vi "Get System Properties.vi"(8 "error in (no error)":errorcluster, 11 "RT System Monitor in":refnum<class "RT System Monitor.lvclass">) -> (0 "error out":errorcluster, 2 "System Health Data":T1 {"Hard Drive Space Used (%)" scale=0.0..100.0}, 3 "RT System Monitor out":refnum<class "RT System Monitor.lvclass">)   [LabVIEW 2017, in "RT System Monitor.lvclass"]
doc: "Poll for CPU usage properties.\nGet total physical memory, hard drive capacity, and total virtual memory.\nPoll for free physical memory, free hard drive space, largest contiguous block of memory, and free virtual memory."
uses:
  RT System Monitor.lvclass
  Shared/System Health Data.ctl
  RT System Monitor.lvclass/RT System Monitor.ctl
  <resource>/objmgr/nicriosae.rc
  <resource>/objmgr/nisysapi.rc
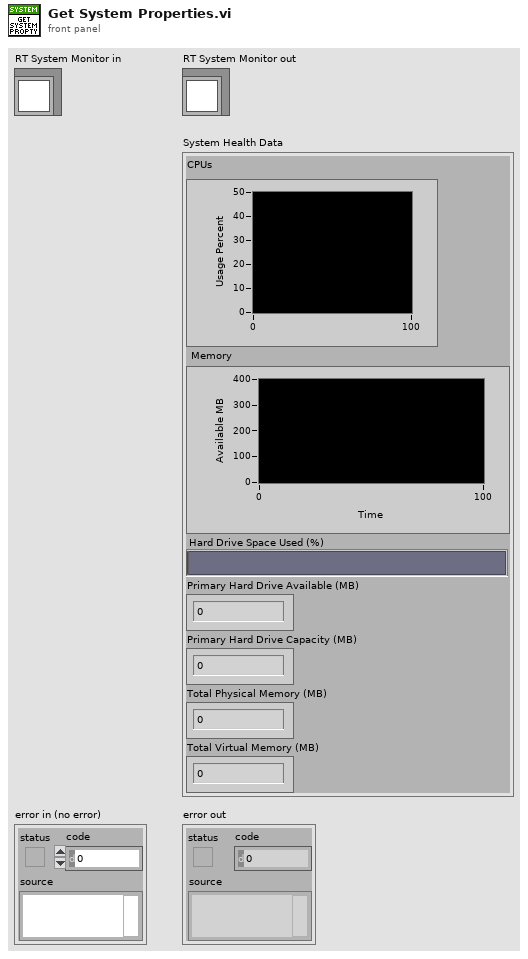
[diagram p1: front panel]
types:
  T1 = typedef "System Health Data.ctl" = cluster{"CPUs":u32[][], "Memory":dbl[][], "Hard Drive Space Used (%)":dbl, "Primary Hard Drive Available (MB)":dbl, "Primary Hard Drive Capacity (MB)":u32, "Total Physical Memory (MB)":u32, "Total Virtual Memory (MB)":u32}
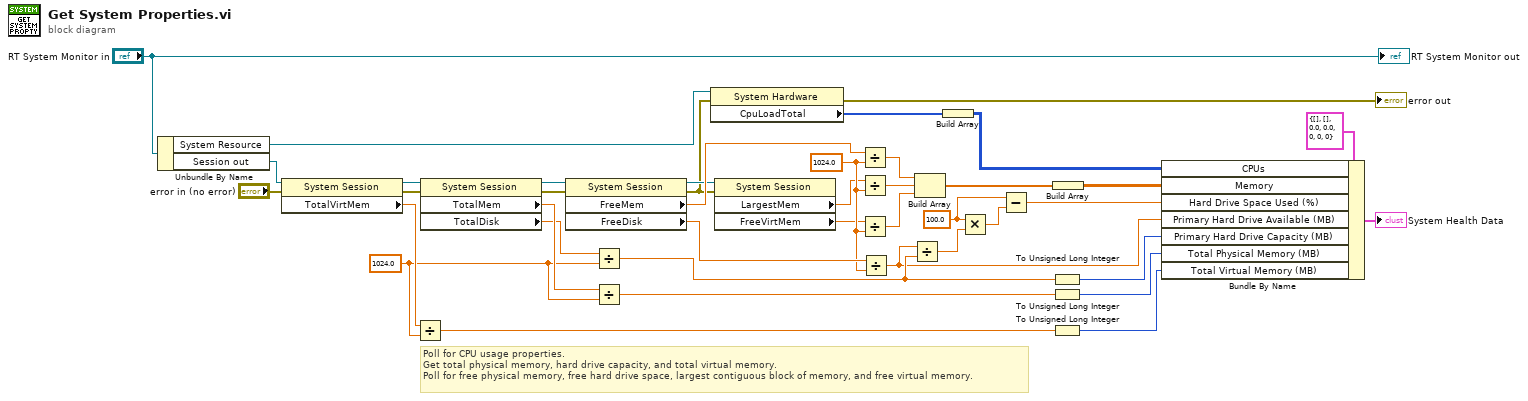
[diagram p0: block diagram]
diagram:
  w19 = 100.0 ("y")
  w24 = 1024.0
  w37 = 1024.0
  # "Poll for CPU usage properties.\nGet total physical memory, hard drive capacity, and total virtual memory.\nPoll for free physical memory, free hard drive space, largest contiguous block of memory, and free virtual memory."
  n1 = Unbundle By Name("RT System Monitor in") -> ("System Resource"=w4:refnum<k20>, "Session out"=w30:refnum<k21>)
  n2 = property class="System Session"(reference=w30, error in="error in (no error)") -> (reference out=w6:refnum<k21>, error out=w13:errorcluster, "TotalVirtMem"=w38:dbl)
  n3 = Divide(x=w38, y=w37) -> (x/y=w35:dbl)
  n4 = property class="System Session"(reference=w6, error in=w13) -> (reference out=w34:refnum<k21>, error out=w32:errorcluster, "TotalMem"=w40:dbl, "TotalDisk"=w39:dbl)
  n5 = property class="System Session"(reference=w34, error in=w32) -> (reference out=w5:refnum<k21>, error out=w3:errorcluster, "FreeMem"=w29:dbl, "FreeDisk"=w25:dbl)
  n6 = Divide(x=w39, y=w37) -> (x/y=w33:dbl)
  n7 = Divide(x=w40, y=w37) -> (x/y=w36:dbl)
  n8 = property class="System Hardware"(reference=w4, error in=w3) -> (error out=→"error out":errorcluster, "CpuLoadTotal"=w2:u32[])  [unwired: 1 out]
  n9 = property class="System Session"(reference=w5, error in=w3) -> ("LargestMem"=w21:dbl, "FreeVirtMem"=w22:dbl)  [unwired: 2 out]
  n10 = Divide(x=w29, y=w24) -> (x/y=w27:dbl)
  n11 = Divide(x=w21, y=w24) -> (x/y=w26:dbl)
  n12 = Divide(x=w22, y=w24) -> (x/y=w23:dbl)
  n13 = Divide(x=w25, y=w24) -> (x/y=w10:dbl)
  n14 = Divide(x=w10, y=w33) -> (x/y=w18:dbl)
  n15 = Build Array(w27, w26, w23) -> (w28:dbl[])
  n16 = Build Array(w2) -> (w1:u32[][])
  n17 = Multiply(x=w19, y=w18) -> (x*y=w20:dbl)
  n18 = Subtract(x=w19, y=w20) -> (x-y=w14:dbl)
  n19 = To Unsigned Long Integer(number=w33) -> (unsigned 32bit integer=w9:u32)
  n20 = To Unsigned Long Integer(number=w36) -> (unsigned 32bit integer=w8:u32)
  n21 = To Unsigned Long Integer(number=w35) -> (unsigned 32bit integer=w7:u32)
  n22 = Build Array(w28) -> (w15:dbl[][])
  n23 = Bundle By Name(cluster=T1 {"CPUs"=[], "Memory"=[], "Hard Drive Space Used (%)"=0.0, "Primary Hard Drive Available (MB)"=0.0, "Primary Hard Drive Capacity (MB)"=0, "Total Physical Memory (MB)"=0, "Total Virtual Memory (MB)"=0} ("System Health Data"), "CPUs"=w1, "Memory"=w15, "Hard Drive Space Used (%)"=w14, "Primary Hard Drive Available (MB)"=w10, "Primary Hard Drive Capacity (MB)"=w9, "Total Physical Memory (MB)"=w8, "Total Virtual Memory (MB)"=w7) -> (→"System Health Data":T1)
  "RT System Monitor out" <- "RT System Monitor in"
